vi "Handle Error.vi"(7 "Stop on Unhandled Error (T)":bool=TRUE, 8 "error in":errorcluster, 11 "DAQmx":refnum<class "DAQmx.lvclass">) -> (0 "handling error":errorcluster, 2 "Unhandled error":errorcluster, 3 "DAQmx out":refnum<class "DAQmx.lvclass">)   [LabVIEW 2019, in "DAQmx.lvclass"]
doc: "JKI State Machine Objects (SMO) 1.0.0.11\nJKI - JKI\nCopyright (c) 2016, JKI"
uses:
  DAQmx.lvclass
  <vilib>/JKI/JKI SMO/SMO/SMO.lvclass
panel:
  # "For instructions on how to use the JKI State Machine Objects, examples and video tutorials, visit:\nhttp://jki.net/state-machine-objects/\n\nJKI State Machine Objects™\nhttp://jki.net/state-machine-objects/\nCopyright (C) 2005-2015, JKI <info@jki.net>\nALL RIGHTS RESERVED"
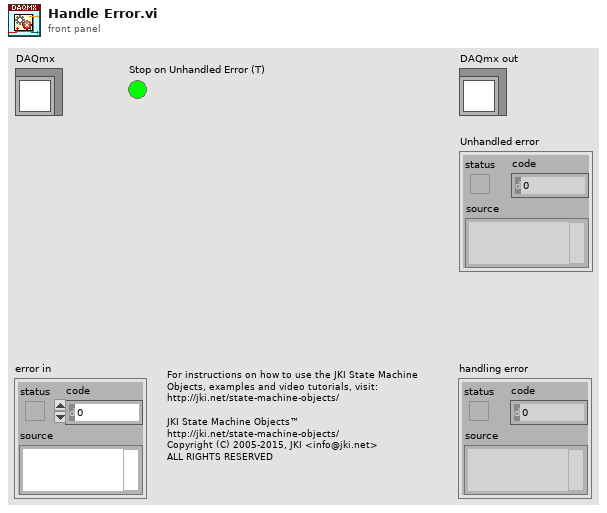
[diagram p1: front panel]
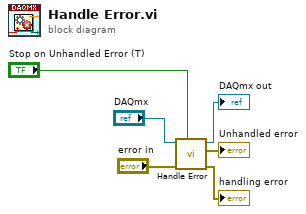
[diagram p0: block diagram]
diagram:
  n1 = call-parent "Handle Error.vi"("Stop on Unhandled Error (T)"="Stop on Unhandled Error (T)", "error in"="error in", "SMO"="DAQmx") -> ("handling error"=→"handling error":errorcluster, "Unhandled error"=→"Unhandled error":errorcluster, "SMO out"=→"DAQmx out":refnum<class "DAQmx.lvclass">)  [unwired: 6 in]
